vi "myTemp Basic Example.vi"() -> ()   [LabVIEW 2013]
panel:
  out "Temperature Datea":cluster{dbl[], dbl[]}[](graph)
  in  "device name":tag="myDAQ1" caption="device name (myDAQ 1)"
  in  "Measurement Loop Time":i32=1 min=1 max=10000 step=1 format="%#.3f sec"
  in  "myTemp Setup":T1={"Offset Temp"=0.0, "Set Offset"=FALSE, "Calibration Data"=[{"Ka"=0.000739984, "Kb"=0.000278736, "Kc"=9.26322e-08}, {"Ka"=0.00073998, "Kb"=0.00027874, "Kc"=9.2632e-08}, {"Ka"=0.00073998, "Kb"=0.00027874, "Kc"=9.2632e-08}, {"Ka"=0.00073998, "Kb"=0.00027874, "Kc"=9.2632e-08}, {"Ka"=0.00073998, "Kb"=0.00027874, "Kc"=9.2632e-08}, {"Ka"=0.00073998, "Kb"=0.00027874, "Kc"=9.2632e-08}, {"Ka"=0.00073998, "Kb"=0.00027874, "Kc"=9.2632e-08}], "Chan Select"=[TRUE, TRUE, TRUE, FALSE, FALSE, FALSE, FALSE], "Clear Offsets"=FALSE, "Input Mode"=FALSE, "Chart History Length"=2000, "Use One K Set"=TRUE} {"Chart History Length" min=1 max=10000 step=1; "Calibration Data"."Kc" format="%#.4e"; "Calibration Data"."Kb" format="%#.4e"; "Calibration Data"."Ka" format="%#.4e"; "Offset Temp" min=-40.0 max=250.0 step=1.0}
  out "Thermometers":dbl[](array[slide]) scale=0.0..100.0 scale format="%#.2f"
  in  "stop":bool
  # "PITSCO myTemp - Temperature Measurement Example"
  # "<<< Scroll left to see/change measurement settings"
  # "Select Temperature Channels to Display"
  # "Temp1"
  # "Temp2"
  # "Temp3"
  # "Temp4"
  # "Temp5"
  # "Temp6"
  # "Temp7"
  # "Null Temperature Setting"
  # "Calibration Coefficients"
  # "Temp1"
  # "Temp2"
  # "Temp3"
  # "Temp4"
  # "Temp5"
  # "Temp6"
  # "Temp7"
  # "Ka"
  # "Kb"
  # "Kc"
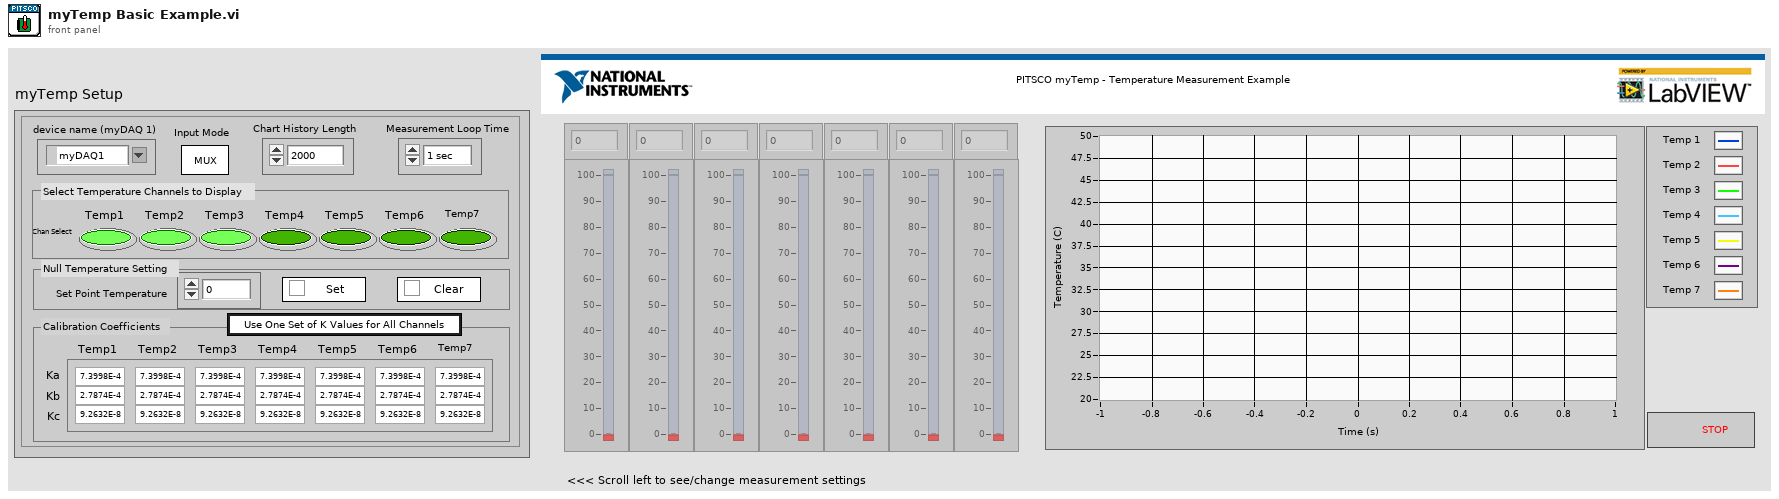
[diagram p1: front panel]
types:
  T1 = cluster{"Offset Temp":dbl, "Set Offset":bool, "Calibration Data":cluster{"Ka":dbl, "Kb":dbl, "Kc":dbl}[], "Chan Select":bool[], "Clear Offsets":bool, "Input Mode":bool, "Chart History Length":i32, "Use One K Set":bool}
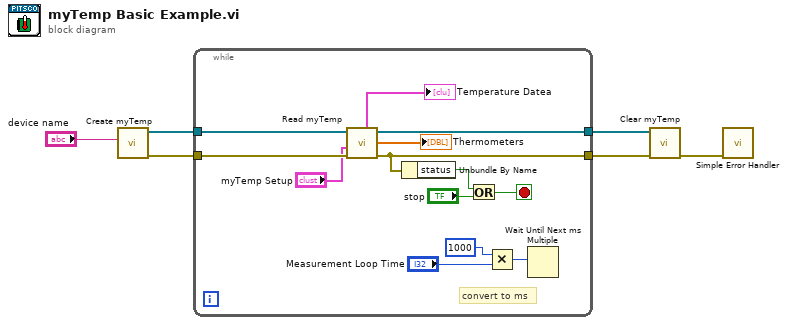
[diagram p0: block diagram]
diagram:
  n1 = call "Create myTemp.vi"("device name (myDAQ1)"="device name") -> ("error out"=w3:errorcluster, "task array out"=w5:refnum<k21>[])  [unwired: 9 in]
  n2 = while {
    tunnel: w5 -> [w16]
    tunnel: w3 -> [w15]
    tunnel: [w14] -> w2
    tunnel: [w13] -> w1
    stop <- w18 stop-if-true
    # "convert to ms"
    n3 = call "Read myTemp.vi"("error in (no error)"=w15, "myTemp Setup"="myTemp Setup", "task array in"=w16) -> ("error out"=w14:errorcluster, "temperature values (°C)"=→"Thermometers":dbl[], "task array out"=w13:refnum<k21>[], "XY Graph"=→"Temperature Datea":cluster{"X":dbl[], "Y":dbl[]}[])  [unwired: 4 in, 1 out]
    n4 = Unbundle By Name(w14) -> ("status"=w17:bool)
    n5 = Or(x=w17, y="stop") -> (x .or. y?=w18:bool)
    n6 = Multiply(x=1000, y="Measurement Loop Time") -> (x*y=w10:i32)
    n7 = Wait Until Next ms Multiple(millisecond multiple=w10) -> ()  [unwired: 1 out]
  }
  n8 = call "Clear myTemp.vi"("error in (no error)"=w2, "task array in"=w1) -> ("error out"=w6:errorcluster)  [unwired: 9 in]
  n9 = call <vilib>:"Simple Error Handler.vi"("error in (no error)"=w6) -> ()  [unwired: 4 in, 5 out]
